vi "PrepareDAQ.vi"(8 "Error in":errorcluster, 9 "BufferTimeout":i32=3000, 11 "DevicesAndSignals":T1) -> (0 "Error out":errorcluster, 2 "DaqMeasurement":refnum<k24>, 3 "DevicesAndSignals":T1)   [LabVIEW 2016]
doc: "Prepares a continuous measurement.\nIf any signal does not belong to the given devices or the device does not support the demanded sample rate, an error will be thrown.\n\nDevicesAndSignals: Array of devices and their signals that have been chosen for measurement\nDaqMeasurement: Reference to the DaqMearurement object that handles the measurement\nBufferTimeout: Buffer timeout in milliseconds (default is 3000ms). Used to calculate size of internal circular buffer. At least there is a buffer of 1000 values for each signal. Normally the buffer size is (bufferTimeout/1000)*sample rate of the signal, prior added to the measurement (E.g.: Signal.SampleRate=1200Hz, bufferTimeOut=1000ms => size of internal circular buffer is 1200 entries)"
uses:
  C:/Users/CL/Desktop/ZcDAQprj0811/ZcDAQprj/Modules/DAQ-Device/Hardware Drivers/QX/HBM LabVIEW Driver/DLLs/Hbm.Api.Common.dll
  DLLs/Hbm.Api.Common.dll
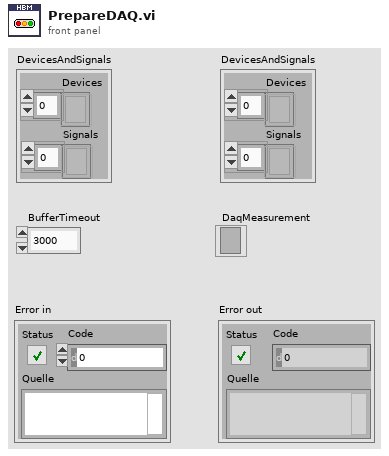
[diagram p1: front panel]
types:
  T1 = cluster{"Devices":refnum<k24>[], "Signals":refnum<k24>[]}
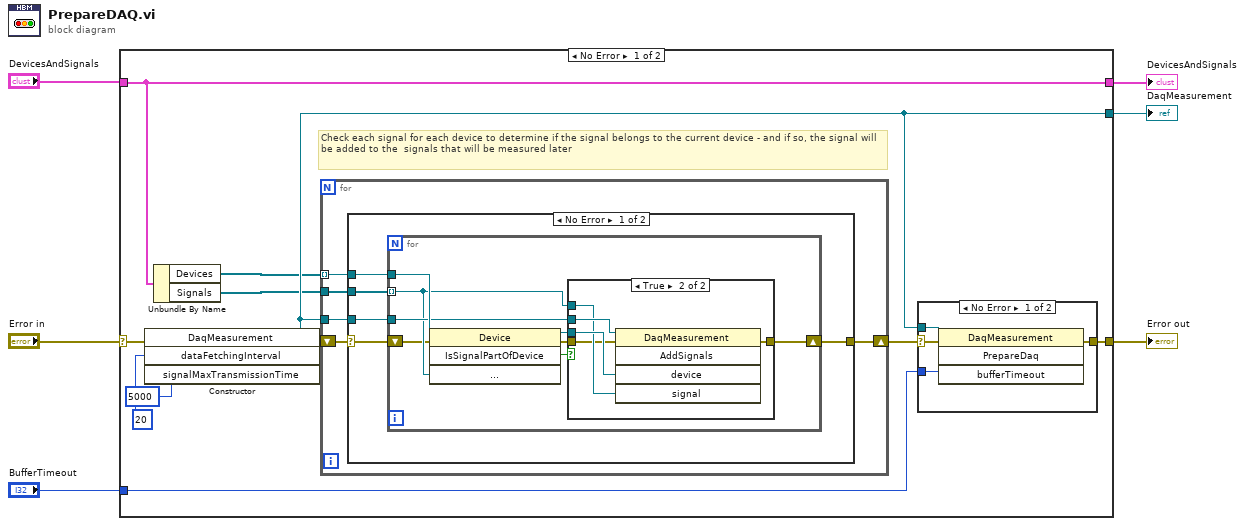
[diagram p0: block diagram]
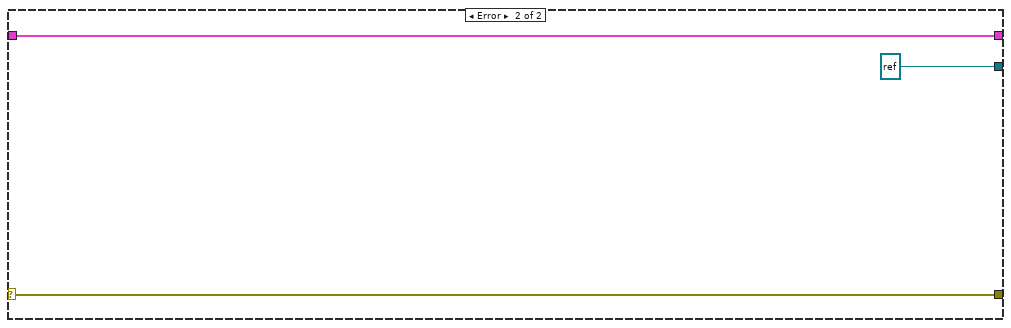
[diagram p5: hidden frame]
diagram:
  n1 = case shown="No Error" "Error in" {
    selector: "Error in" -> [w16 w50]
    tunnel: [w13 w50] -> w6
    tunnel: [w12 refnum<k24> refnum ("new reference")] -> w4
    tunnel: [w10 w48] -> w2
    tunnel: "DevicesAndSignals" -> [w10 w48]
    tunnel: "BufferTimeout" -> [w11 _]
    frame No Error {
      # "Check each signal for each device to determine if the signal belongs to the current device - and if so, the signal will be added to the  signals that will be measured later"
      n2 = constructor class="DaqMeasurement"(error in=w16, "dataFetchingInterval"=20, "signalMaxTransmissionTime"=5000) -> (reference out=w12:refnum<k24>, error out=w15:errorcluster)  [unwired: 2 in, 3 out]
      n3 = Unbundle By Name(w10) -> ("Devices"=w8:refnum<k24>[], "Signals"=w9:refnum<k24>[])
      n4 = for {
        tunnel: w8 -> [w27] mode=indexing
        tunnel: w9 -> [w25]
        tunnel: w12 -> [w26]
        shift-right: [w24] -> w14
        shift-left: w15 -> [w23]
        n5 = case shown="No Error" w23 {
          selector: w23 -> [w28 w47]
          tunnel: w27 -> [w32 _]
          tunnel: w26 -> [w31 _]
          tunnel: w25 -> [w30 _]
          tunnel: [w29 w47] -> w24
          frame No Error {
            n6 = for {
              tunnel: w32 -> [w40]
              tunnel: w31 -> [w38]
              tunnel: w30 -> [w36] mode=indexing
              shift-right: [w34] -> w29
              shift-left: w28 -> [w33]
              n7 = invoke on="Methodenknoten" class="Device" method="IsSignalPartOfDevice"(reference=w40, error in=w33, "signalToCheck"=w36) -> (reference out=w37:refnum<k24>, error out=w35:errorcluster, "IsSignalPartOfDevice"=w39:bool)  [unwired: 1 in, 1 out]
              n8 = case shown="True" w39 {
                tunnel: w38 -> [_ w46]
                tunnel: w37 -> [_ w45]
                tunnel: w36 -> [_ w44]
                tunnel: [w41 w43] -> w34
                tunnel: w35 -> [w41 w42]
                frame False {
                }
                frame True {
                  n9 = invoke on="Methodenknoten" class="DaqMeasurement" method="AddSignals"(reference=w46, error in=w42, "device"=w45, "signal"=w44) -> (error out=w43:errorcluster)  [unwired: 1 in, 4 out]
                }
              }
            }
          }
          frame Error {
          }
        }
      }
      n10 = case shown="No Error" w14 {
        selector: w14 -> [w20 w22]
        tunnel: [w19 w22] -> w13
        tunnel: w12 -> [w21 _]
        tunnel: w11 -> [w18 _]
        frame No Error {
          n11 = invoke on="Methodenknoten" class="DaqMeasurement" method="PrepareDaq"(reference=w21, error in=w20, "bufferTimeout"=w18) -> (error out=w19:errorcluster)  [unwired: 1 in, 3 out]
        }
        frame Error {
        }
      }
    }
    frame Error {
    }
  }
  "Error out" <- w6
  "DaqMeasurement" <- w4
  "DevicesAndSignals" <- w2
